vi "SVT Sound Level (1 Ch).vi"(0 "scaled signal [EU]":waveform(dbl), 1 "integration time [s]":dbl=1.0 format="%.2f", 5 "measurement selection":T1={"Leq"=TRUE, "Running Leq"=FALSE, "Exponential"=FALSE, "Peak"=FALSE}, 7 "exponential mode":enum16{"Slow", "Fast", "Impulse", "Custom"}(ring)=enum."Fast", 9 "time constant [ms]":dbl=125.0 format="%.2f", 11 "error in (no error)":errorcluster, 12 "restart averaging (F)":bool) -> (3 "exp avg sound level [dB EU]":waveform(dbl), 4 "Leq sound level [dB EU]":waveform(dbl), 6 "running Leq sound level [dB EU]":waveform(dbl), 8 "peak sound level [dB pk EU]":waveform(dbl), 14 "unit label":string, 15 "error out":errorcluster)   [LabVIEW 2017, in "SoundVib_SoundLevel.lvlib"]
doc: "Computes several sound level measurements including equivalent continuous level (Leq), running Leq sound levels, exponential averaged sound level, and the peak sound level. Wire data to the <B>scaled signal [EU]</B> input to determine the polymorphic instance to use or manually select the instance."
uses:
  <vilib>/addons/Sound and Vibration/svt_Level/SoundVib_SoundLevel.lvlib
  <vilib>/addons/Sound and Vibration/svt_Level/SVL Peak Sound Level (1 Ch).vi
  <vilib>/addons/Sound and Vibration/svt_Level/SVL Decimated Exp Avg Sound Level (1 Ch).vi
  <vilib>/addons/Sound and Vibration/svt_Level/SVL Running Leq Sound Level (1 Ch).vi
  <vilib>/addons/Sound and Vibration/svt_Level/SVL Leq Sound Level (1 Ch).vi
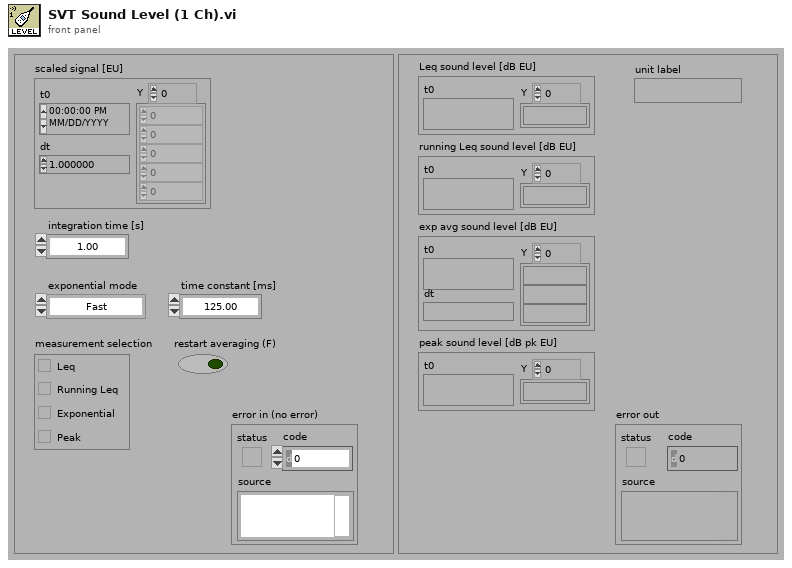
[diagram p1: front panel]
types:
  T1 = cluster{"Leq":bool, "Running Leq":bool, "Exponential":bool, "Peak":bool}
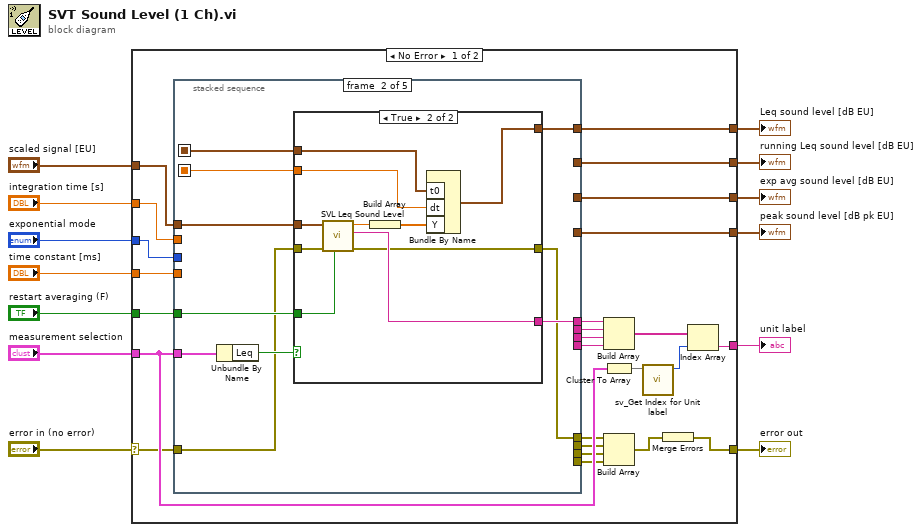
[diagram p0: block diagram]
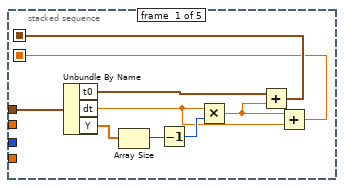
[diagram p2: hidden frame]
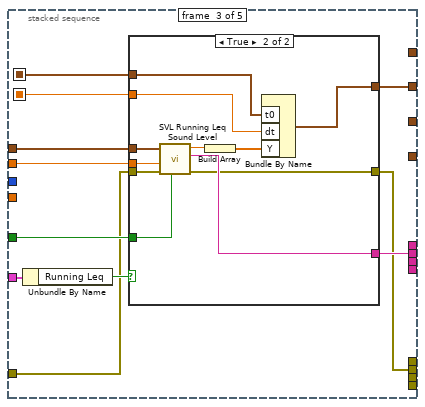
[diagram p4: hidden frame]
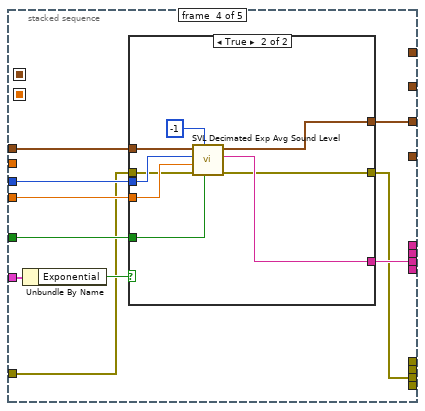
[diagram p6: hidden frame]
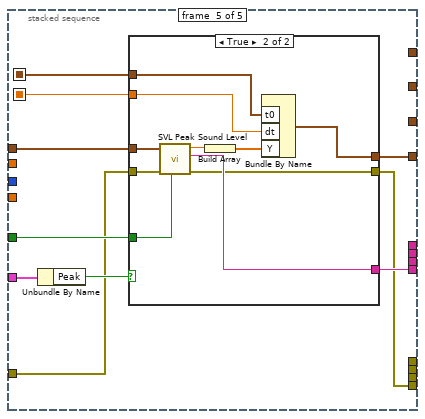
[diagram p8: hidden frame]
diagram:
  n1 = case shown="No Error" "error in (no error)" {
    selector: "error in (no error)" -> [w18 w133]
    tunnel: "scaled signal [EU]" -> [w38 _]
    tunnel: "restart averaging (F)" -> [w37 _]
    tunnel: [w36 _] -> w11
    tunnel: [w35 _] -> w10
    tunnel: "integration time [s]" -> [w34 _]
    tunnel: "exponential mode" -> [w33 _]
    tunnel: "time constant [ms]" -> [w32 _]
    tunnel: [w31 _] -> w6
    tunnel: [w30 _] -> w5
    tunnel: "measurement selection" -> [w29 _]
    tunnel: [w14 _] -> w3
    tunnel: [w19 w133] -> w2
    frame No Error {
      n2 = stacked-sequence {
        seq-local: [w39 _ _ _ _] -> [_ w52 w74 _ w116]
        seq-local: [w42 _ _ _ _] -> [_ w53 w75 _ w117]
        tunnel: w29 -> [_ w57 w79 w101 w121]
        tunnel: w38 -> [w47 w55 w77 w99 w119]
        tunnel: w37 -> [_ w54 w76 w98 w118]
        tunnel: [_ w51 _ _ _] -> w36
        tunnel: [_ _ w73 _ _] -> w35
        tunnel: w34 -> [_ _ w72 _ _]
        tunnel: w33 -> [_ _ _ w97 _]
        tunnel: w32 -> [_ _ _ w96 _]
        tunnel: [_ _ _ w95 _] -> w31
        tunnel: [_ _ _ _ w115] -> w30
        tunnel: [_ w50 _ _ _] -> w28
        tunnel: [_ _ w71 _ _] -> w27
        tunnel: [_ _ _ w94 _] -> w26
        tunnel: [_ _ _ _ w114] -> w25
        tunnel: w18 -> [_ w49 w70 w93 w113]
        tunnel: [_ w48 _ _ _] -> w24
        tunnel: [_ _ w69 _ _] -> w23
        tunnel: [_ _ _ w92 _] -> w22
        tunnel: [_ _ _ _ w112] -> w21
        frame #0 {
          n3 = Unbundle By Name(w47) -> ("t0"=w44:timestamp, "dt"=w40:dbl, "Y"=w46:dbl[])
          n4 = Array Size(array=w46) -> (size(s)=w45:i32)
          n5 = Decrement(x=w45) -> (x-1=w43:i32)
          n6 = Multiply(x=w40, y=w43) -> (x*y=w41:dbl)
          n7 = Add(x=w44, y=w41) -> (x+y=w42:timestamp)
          n8 = Add(x=w41, y=w40) -> (x+y=w39:dbl)
        }
        frame #1 {
          n9 = Unbundle By Name(w57) -> ("Leq"=w56:bool)
          n10 = case shown="True" w56 {
            tunnel: w55 -> [_ w68]
            tunnel: w54 -> [_ w67]
            tunnel: w53 -> [_ w64]
            tunnel: w52 -> [_ w63]
            tunnel: [_ w62] -> w51
            tunnel: [_ w61] -> w50
            tunnel: w49 -> [w58 w60]
            tunnel: [w58 w59] -> w48
            frame False {
            }
            frame True {
              n11 = call-poly <vilib>:"SVL Leq Sound Level.vi"("restart averaging (F)"=w67, "error in (no error)"=w60, "scaled signal [EU]"=w68) -> ("error out"=w59:errorcluster, "unit label"=w61:string, "Leq sound level [dB EU]"=w66:dbl)  [unwired: 6 in]
              n12 = Build Array(w66) -> (w65:dbl[])
              n13 = Bundle By Name("t0"=w64, "dt"=w63, "Y"=w65) -> (w62:waveform(dbl))  [unwired: 1 in]
            }
          }
        }
        frame #2 {
          n14 = Unbundle By Name(w79) -> ("Running Leq"=w78:bool)
          n15 = case shown="True" w78 {
            tunnel: w77 -> [_ w88]
            tunnel: w76 -> [_ w87]
            tunnel: w75 -> [_ w90]
            tunnel: w74 -> [_ w89]
            tunnel: [_ w85] -> w73
            tunnel: w72 -> [_ w84]
            tunnel: [_ w83] -> w71
            tunnel: w70 -> [w80 w82]
            tunnel: [w80 w81] -> w69
            frame False {
            }
            frame True {
              n16 = call-poly <vilib>:"SVL Running Leq Sound Level.vi"("restart averaging (F)"=w87, "error in (no error)"=w82, "integration time [s]"=w84, "scaled signal [EU]"=w88) -> ("error out"=w81:errorcluster, "unit label"=w83:string, "running Leq sound level [dB EU]"=w86:dbl)  [unwired: 4 in, 1 out]
              n17 = Build Array(w86) -> (w91:dbl[])
              n18 = Bundle By Name("t0"=w90, "dt"=w89, "Y"=w91) -> (w85:waveform(dbl))  [unwired: 1 in]
            }
          }
        }
        frame #3 {
          n19 = Unbundle By Name(w101) -> ("Exponential"=w100:bool)
          n20 = case shown="True" w100 {
            tunnel: w99 -> [_ w111]
            tunnel: w98 -> [_ w110]
            tunnel: w97 -> [_ w109]
            tunnel: w96 -> [_ w108]
            tunnel: [_ w106] -> w95
            tunnel: [_ w105] -> w94
            tunnel: w93 -> [w102 w104]
            tunnel: [w102 w103] -> w92
            frame False {
            }
            frame True {
              n21 = call-poly <vilib>:"SVL Decimated Exp Avg Sound Level.vi"("restart averaging (F)"=w110, "decimation factor"=-1, "error in (no error)"=w104, "time constant [ms]"=w108, "exponential mode"=w109, "scaled signal [EU]"=w111) -> ("error out"=w103:errorcluster, "unit label"=w105:string, "decimated exp avg sound level [dB EU]"=w106:waveform(dbl))  [unwired: 1 in, 2 out]
            }
          }
        }
        frame #4 {
          n22 = Unbundle By Name(w121) -> ("Peak"=w120:bool)
          n23 = case shown="True" w120 {
            tunnel: w119 -> [_ w129]
            tunnel: w118 -> [_ w128]
            tunnel: w117 -> [_ w131]
            tunnel: w116 -> [_ w130]
            tunnel: [_ w126] -> w115
            tunnel: [_ w125] -> w114
            tunnel: w113 -> [w122 w124]
            tunnel: [w122 w123] -> w112
            frame False {
            }
            frame True {
              n24 = call-poly <vilib>:"SVL Peak Sound Level.vi"("restart averaging (F)"=w128, "error in (no error)"=w124, "scaled signal [EU]"=w129) -> ("error out"=w123:errorcluster, "unit label"=w125:string, "peak sound level [dB pk EU]"=w127:dbl)  [unwired: 6 in]
              n25 = Build Array(w127) -> (w132:dbl[])
              n26 = Bundle By Name("t0"=w131, "dt"=w130, "Y"=w132) -> (w126:waveform(dbl))  [unwired: 1 in]
            }
          }
        }
      }
      n27 = Build Array(w28, w27, w26, w25) -> (w16:string[])
      n28 = Cluster To Array(cluster=w29) -> (array=w17:bool[])
      n29 = Build Array(w24, w23, w22, w21) -> (w20:errorcluster[])
      n30 = call <vilib>:"sv_Get Index for Unit label.vi"("measurement selection"=w17) -> ("index"=w15:i32)  [unwired: 10 in]
      n31 = Merge Errors(w20) -> (w19:errorcluster)
      n32 = Index Array(array=w16, index=w15) -> (element=w14:string)
    }
    frame Error {
    }
  }
  "error out" <- w2
  "exp avg sound level [dB EU]" <- w6
  "Leq sound level [dB EU]" <- w11
  "running Leq sound level [dB EU]" <- w10
  "peak sound level [dB pk EU]" <- w5
  "unit label" <- w3
